vi "1.2.vi"() -> ()   [LabVIEW 2020]
panel:
  out "String":string
  in  "Hello there!":string
  out "XOR":bool
  in  "B":bool
  in  "A":bool
  in  "kPa":dbl
  out "Gauge":dbl(knob) scale=0.0..10.0
  out "Thermometer":dbl(slide) scale=0.0..100.0
  in  "Temperatura":dbl
  out "¿Cual es la mejor carrera xd?":string
  in  "Carrera":string
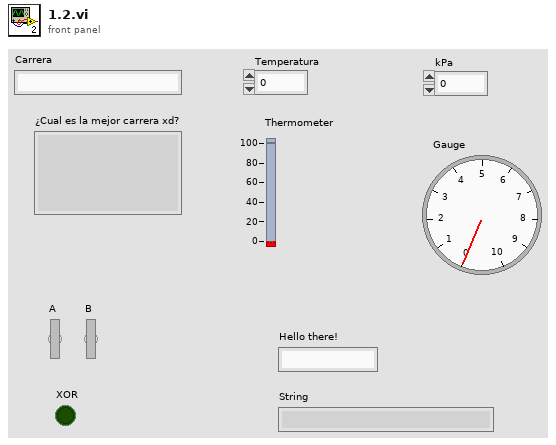
[diagram p1: front panel]
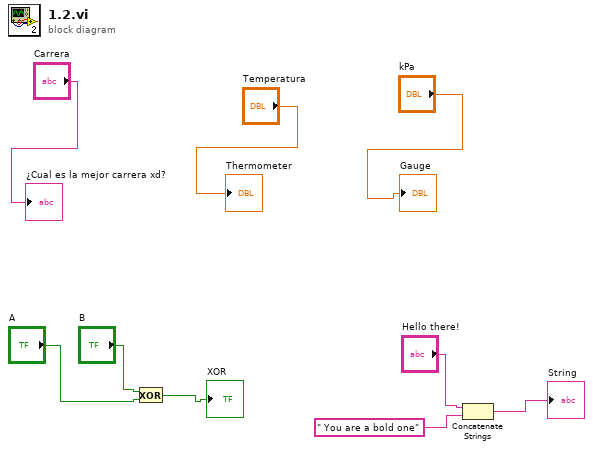
[diagram p0: block diagram]
diagram:
  n1 = Exclusive Or(1:"A", 2:"B") -> (0:→"XOR":bool)
  n2 = Concatenate Strings("Hello there!", " You are a bold one") -> (→"String":string)
  "¿Cual es la mejor carrera xd?" <- "Carrera"
  "Thermometer" <- "Temperatura"
  "Gauge" <- "kPa"
